vi "SubMenu.vi"(4 "ContextMenu":bool, 6 "SubMenu":bool, 7 "User Event":refnum<user-event>, 8 "error in (no error)":errorcluster, 9 "Tag":string, 10 "Selected Area":T2, 11 "Menu in":refnum<class "Menu.lvclass">) -> (0 "error out":errorcluster, 3 "Menu out":refnum<class "Menu.lvclass">)   [LabVIEW 2021, in "Menu.lvlib" / "Menu.lvclass"]
uses:
  Menu.lvclass
  <vilib>/Utility/miscctls.llb/LVPoint32TypeDef.ctl
  <vilib>/Utility/miscctls.llb/LVRectTypeDef.ctl
  <vilib>/event_ctls.llb/usereventprio.ctl
  UIShadow/src/Shadow.lvclass
  <vilib>/Utility/miscctls.llb/LVPositionTypeDef.ctl
  MenuSelection.ctl
  dc479f3e-3cf5-4ae2-bb41-5e206b11c71e.vi
  GetBackgroundColor.vi
  GetDVR.vi
  Picture2D/src/Color/Color.lvclass
  Menu.lvclass/Menu.ctl
  FrontPanel/src/FrontPanel.lvlib
panel:
  in  "Coords":T1
  in  "CtrlRef":refnum<vi>
  in  "notifier":refnum<notifier>
  out "Selected Area":T2
  out "Selected Tag":string
  out "Picture":picture
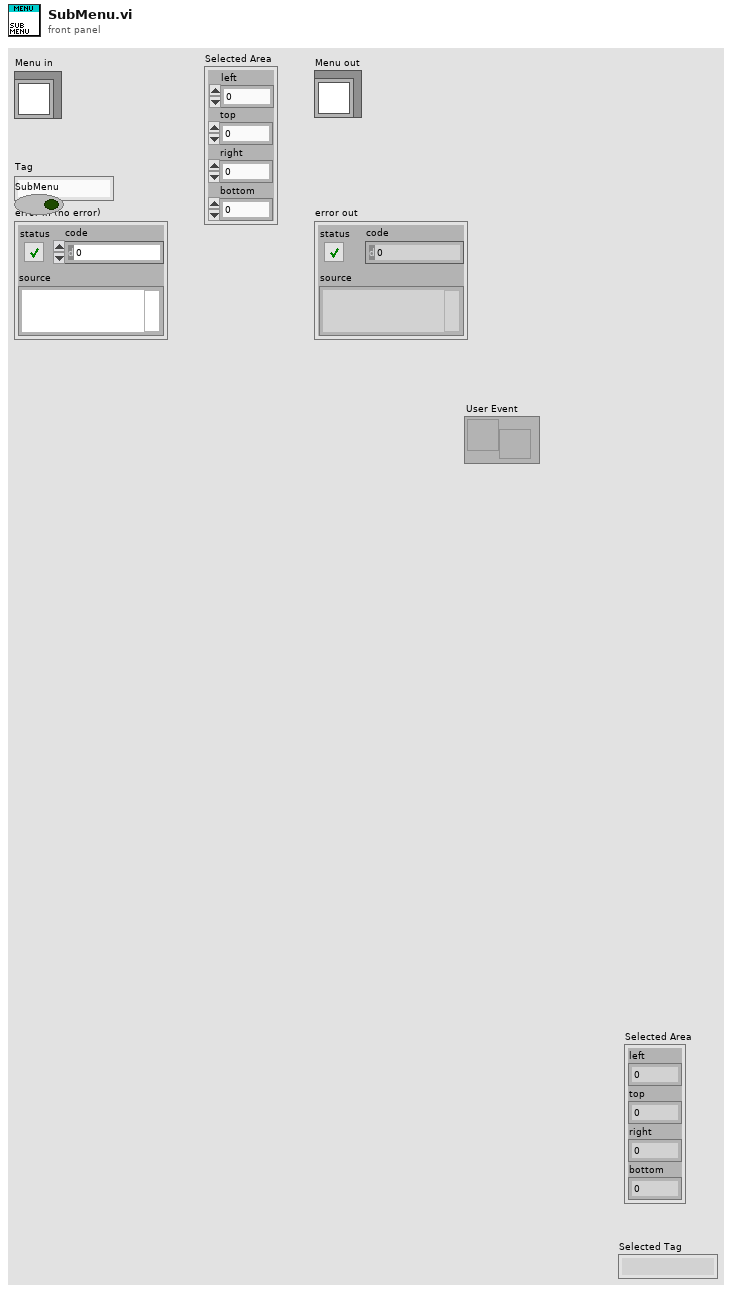
[diagram p1: front panel]
types:
  T1 = typedef "LVPoint32TypeDef.ctl" = cluster{"Horizontal":i32, "Vertical":i32}
  T2 = cluster{"left":i16, "top":i16, "right":i16, "bottom":i16}
  T3 = typedef "LVRectTypeDef.ctl" = cluster{"Left":i16, "Top":i16, "Right":i16, "Bottom":i16}
  T4 = typedef "usereventprio.ctl" = enum32{"high priority", "normal priority"}
  T5 = typedef "LVPositionTypeDef.ctl" = cluster{"Left":i32, "Top":i32}
  T6 = typedef "Menu.lvlib/Menu.lvclass/MenuSelection.ctl" = cluster{"ItemTag":string, "ItemPath":string}
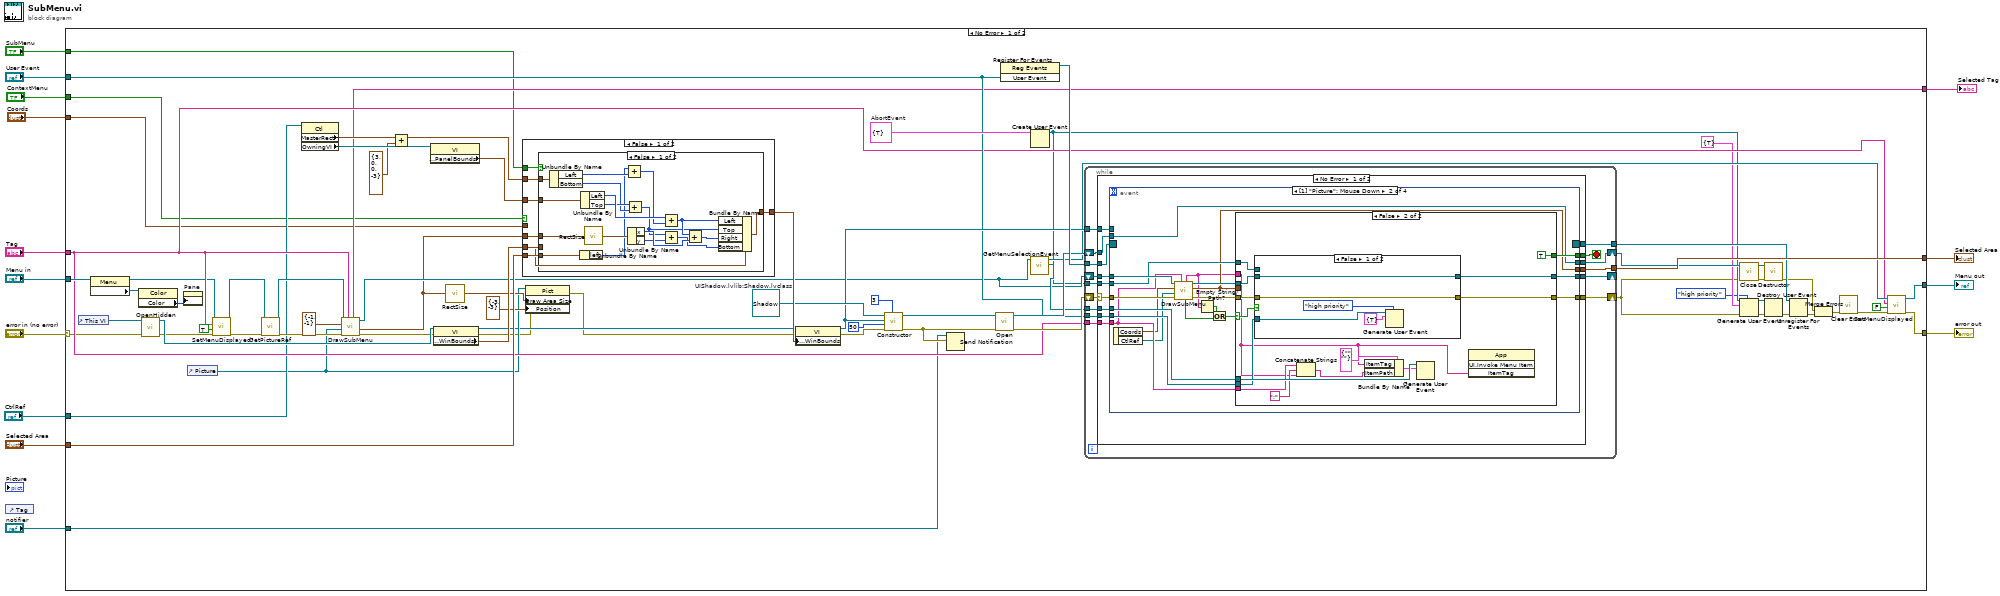
[diagram p0: block diagram]
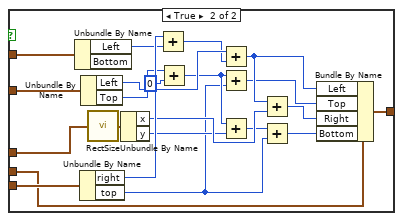
[diagram p2: hidden frame]
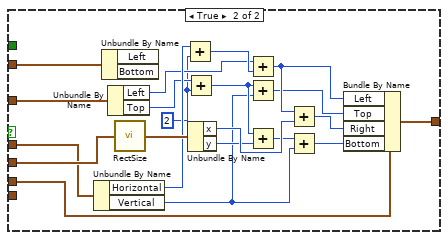
[diagram p3: hidden frame]
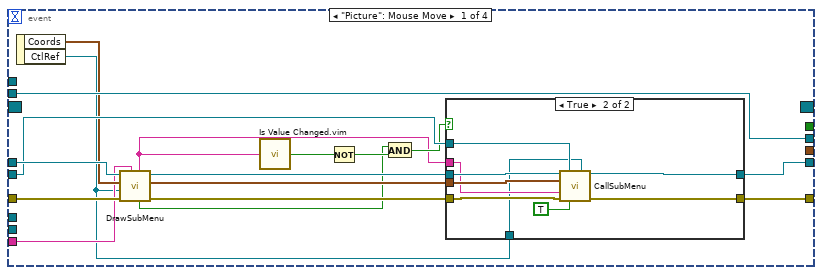
[diagram p4: hidden frame]
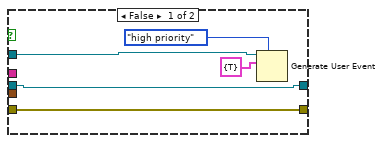
[diagram p5: hidden frame]
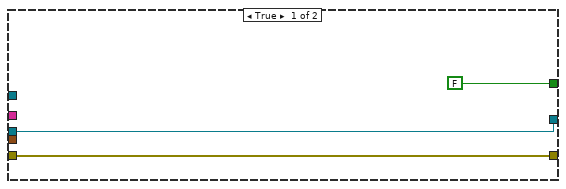
[diagram p6: hidden frame]
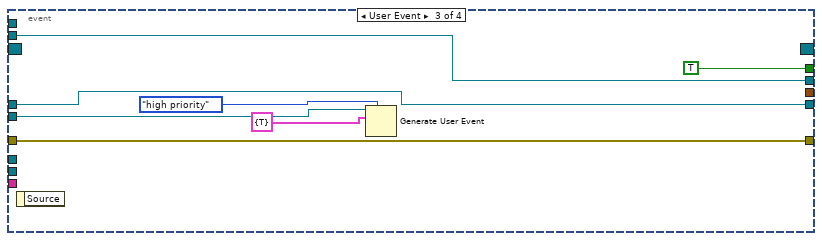
[diagram p8: hidden frame]
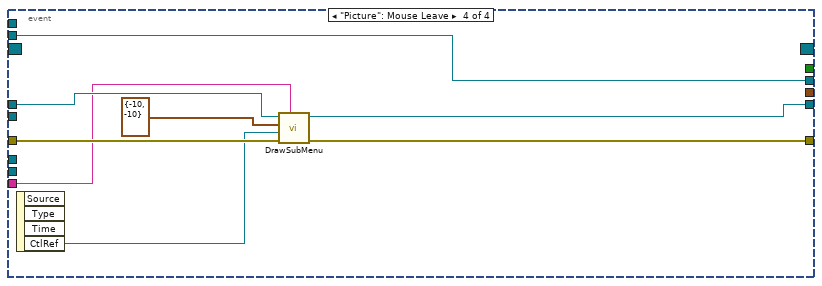
[diagram p9: hidden frame]
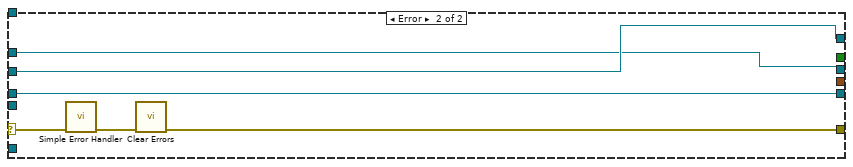
[diagram p10: hidden frame]
diagram:
  n1 = control-ref of="Tag"() -> ()  [unwired: 1 out]
  n2 = case shown="No Error" "error in (no error)" {
    selector: "error in (no error)" -> [w42 w281]
    tunnel: "Selected Area" -> [w84 _]
    tunnel: [w77 _] -> w13
    tunnel: "SubMenu" -> [w28 _]
    tunnel: "User Event" -> [w58 _]
    tunnel: "Menu in" -> [w55 w282]
    tunnel: [w51 w282] -> w9
    tunnel: "Tag" -> [w50 _]
    tunnel: [w48 w281] -> w7
    tunnel: "notifier" -> [w30 _]
    tunnel: [w29 _] -> w4
    tunnel: "CtrlRef" -> [w23 _]
    tunnel: "ContextMenu" -> [w21 _]
    tunnel: "Coords" -> [w20 _]
    frame No Error {
      w70 = refnum<class "Shadow.lvclass"> refnum  # UIShadow.lvlib:Shadow.lvclass
      w74 = cluster{"Abort":bool} {"Abort"=TRUE}  # AbortEvent
      n3 = control-ref of="This VI"() -> (w68:refnum<vi>)
      n4 = property class="Menu"(reference=w55) -> (reference out=w26:refnum<class "Menu.lvclass">, "Public:Background Color"=w25:refnum<class "Color.lvclass">)  [unwired: 1 in, 1 out]
      n5 = property class="Color"(reference=w25) -> ("Color"=w24:u32)  [unwired: 1 in, 2 out]
      n6 = call "OpenHidden.vi"("error in (no error)"=w42, "VI in"=w68) -> ("error out"=w41:errorcluster, "VI out"=w85:refnum<vi>)  [unwired: 8 in]
      n7 = property on="Pane" class="Pane"("PaneColor"=w24) -> ()  [unwired: 2 in, 2 out]
      n8 = control-ref of="Picture"() -> (w22:refnum<vi>)
      n9 = call "SetMenuDisplayed.vi"("error in (no error)"=w41, "Displayed"=TRUE, "Tag"=w50, "Menu in"=w26) -> ("error out"=w47:errorcluster, "Menu out"=w46:refnum<class "Menu.lvclass">)  [unwired: 6 in]
      n10 = call "GetPictureRef.vi"("error in (no error)"=w47, "Menu in"=w46) -> ("error out"=w44:errorcluster, "Menu out"=w45:refnum<class "Menu.lvclass">)  [unwired: 7 in, 1 out]
      n11 = property class="Ctl"(reference=w23) -> ("MasterRect"=w83:T3, "OwningVI"=w82:refnum<vi>)  [unwired: 1 in, 2 out]
      n12 = call "DrawSubMenu.vi"("Tag"=w50, "error in (no error)"=w44, "Pict Refnum"=w22, "Coords"=T1 {"Horizontal"=-1, "Vertical"=-1}, "Menu in"=w45) -> ("error out"=w43:errorcluster, "Global Area"=w27:T2, "Menu out"=w56:refnum<class "Menu.lvclass">, "Selected Tag"=w29:string)  [unwired: 1 in, 2 out]
      n13 = Add(x=w83, y=T3 {"Left"=3, "Top"=0, "Right"=0, "Bottom"=-3}) -> (x+y=w19:T3)
      n14 = property class="VI"(reference=w82) -> ("Front Panel.PanelBounds"=w81:T3)  [unwired: 1 in, 2 out]
      n15 = property class="VI"(reference=w85, error in=w43) -> (reference out=w17:refnum<vi>, error out=w16:errorcluster, "Front Panel.WinBounds"=w78:T3)
      n16 = call <vilib>:"RectSize.vi"("rect"=w27) -> ("point"=w76:cluster{"x":i16, "y":i16})
      n17 = case shown="False" w21 {
        tunnel: w84 -> [w92 _]
        tunnel: w19 -> [w91 w154]
        tunnel: w81 -> [w90 w153]
        tunnel: [w89 w152] -> w79
        tunnel: w78 -> [w88 w151]
        tunnel: w28 -> [w87 _]
        tunnel: w27 -> [w86 w150]
        tunnel: w20 -> [_ w136]
        frame False {
          n18 = case shown="False" w87 {
            tunnel: w92 -> [w110 w132]
            tunnel: w91 -> [w99 w120]
            tunnel: w90 -> [w98 w119]
            tunnel: [w96 w118] -> w89
            tunnel: w88 -> [w95 w117]
            tunnel: w86 -> [w94 w116]
            frame False {
              n19 = Unbundle By Name(w99) -> ("Left"=w100:i16, "Bottom"=w97:i16)
              n20 = Unbundle By Name(w110) -> ("left"=w93:i16)
              n21 = Unbundle By Name(w98) -> ("Left"=w109:i16, "Top"=w108:i16)
              n22 = call <vilib>:"RectSize.vi"("rect"=w94) -> ("point"=w111:cluster{"x":i16, "y":i16})
              n23 = Add(x=w93, y=w100) -> (x+y=w101:i16)
              n24 = Add(x=w108, y=w97) -> (x+y=w102:i16)
              n25 = Unbundle By Name(w111) -> ("x"=w106:i16, "y"=w103:i16)
              n26 = Add(x=w109, y=w101) -> (x+y=w107:i16)
              n27 = Add(x=w102, y=w103) -> (x+y=w104:i16)
              n28 = Add(x=w107, y=w106) -> (x+y=w105:i16)
              n29 = Bundle By Name(cluster=w95, "Left"=w107, "Top"=w102, "Right"=w105, "Bottom"=w104) -> (w96:T3)
            }
            frame True {
              n30 = Unbundle By Name(w120) -> ("Left"=w121:i16)  [unwired: 1 out]
              n31 = Unbundle By Name(w132) -> ("right"=w130:i16, "top"=w113:i16)
              n32 = Unbundle By Name(w119) -> ("Left"=w131:i16, "Top"=w129:i16)
              n33 = call <vilib>:"RectSize.vi"("rect"=w116) -> ("point"=w133:cluster{"x":i16, "y":i16})
              n34 = Unbundle By Name(w133) -> ("x"=w127:i16, "y"=w124:i16)
              n35 = Add(x=w130, y=w121) -> (x+y=w122:i16)
              n36 = Add(x=w129, y=i16 0) -> (x+y=w123:i16)
              n37 = Add(x=w131, y=w122) -> (x+y=w128:i16)
              n38 = Add(x=w123, y=w113) -> (x+y=w115:i16)
              n39 = Add(x=w123, y=w124) -> (x+y=w125:i16)
              n40 = Add(x=w128, y=w127) -> (x+y=w126:i16)
              n41 = Add(x=w125, y=w113) -> (x+y=w114:i16)
              n42 = Bundle By Name(cluster=w117, "Left"=w128, "Top"=w115, "Right"=w126, "Bottom"=w114) -> (w118:T3)
            }
          }
        }
        frame True {
          w134 = i16 2 ("y")
          n43 = Unbundle By Name(w136) -> ("Horizontal"=w148:i32, "Vertical"=w137:i32)
          n44 = Unbundle By Name(w154) -> ()  [unwired: 2 out]
          n45 = Unbundle By Name(w153) -> ("Left"=w135:i16, "Top"=w147:i16)
          n46 = call <vilib>:"RectSize.vi"("rect"=w150) -> ("point"=w149:cluster{"x":i16, "y":i16})
          n47 = Add(x=w148, y=w134) -> (x+y=w140:i32)
          n48 = Add(x=w147, y=w134) -> (x+y=w141:i16)
          n49 = Unbundle By Name(w149) -> ("x"=w145:i16, "y"=w142:i16)
          n50 = Add(x=w135, y=w140) -> (x+y=w146:i32)
          n51 = Add(x=w141, y=w137) -> (x+y=w139:i32)
          n52 = Add(x=w141, y=w142) -> (x+y=w143:i16)
          n53 = Add(x=w146, y=w145) -> (x+y=w144:i32)
          n54 = Add(x=w143, y=w137) -> (x+y=w138:i32)
          n55 = Bundle By Name(cluster=w151, "Left"=w146, "Top"=w139, "Right"=w144, "Bottom"=w138) -> (w152:T3)
        }
      }
      n56 = property class="Pict"(reference=w22, error in=w16, "Draw Area Size"=w76, "Position"=T5 {"Left"=-3, "Top"=-3}) -> (error out=w15:errorcluster)  [unwired: 1 out]
      n57 = property class="VI"(reference=w17, error in=w15, "Front Panel.WinBounds"=w79) -> (reference out=w62:refnum<vi>, error out=w65:errorcluster)
      n58 = call "Constructor.vi"("Offset"=i16 3, "error in (no error)"=w65, "Transparancy"=50, "VI Refnum"=w62, "Shadow in"=w70) -> ("error out"=w31:errorcluster, "Shadow out"=w64:refnum<class "Shadow.lvclass">)  [unwired: 5 in]
      n59 = Send Notification(notification=w31, notifier=w30) -> ()  [unwired: 1 in, 2 out]
      n60 = call "Open.vi"("error in (no error)"=w31, "Shadow in"=w64) -> ("error out"=w66:errorcluster, "Shadow out"=w63:refnum<class "Shadow.lvclass">)  [unwired: 8 in]
      n61 = register-events(w58) -> (reference out=w73:refnum<event-registration>)  [unwired: 2 in, 1 out]
      n62 = call "GetMenuSelectionEvent.vi"("Menu in"=w56) -> ("MenuSelectionEvent"=w57:refnum<user-event>, "Menu out"=w52:refnum<class "Menu.lvclass">)  [unwired: 8 in, 1 out]
      n63 = Create User Event(user event datatype=w74) -> (user event=w36:refnum<user-event>)  [unwired: 1 in, 1 out]
      n64 = while {
        shift-right: [w168] -> w60
        shift-left: w63 -> [w169]
        shift-right: [w166] -> w34
        shift-left: w66 -> [w167]
        shift-right: [w164] -> _
        shift-left: w56 -> [w165]
        tunnel: w50 -> [w163]
        tunnel: w57 -> [w162]
        tunnel: [w160] -> w77
        tunnel: w73 -> [w159]
        tunnel: [w158] -> w71
        tunnel: w36 -> [w157]
        tunnel: w62 -> [w156]
        tunnel: w58 -> [w155]
        stop <- w161 stop-if-true
        n65 = case shown="No Error" w167 {
          selector: w167 -> [w182 w280]
          tunnel: w169 -> [w184 w276]
          tunnel: [w183 w276] -> w168
          tunnel: [w181 w278] -> w166
          tunnel: w165 -> [w180 w275]
          tunnel: [w179 w275] -> w164
          tunnel: w163 -> [w178 _]
          tunnel: w162 -> [w177 _]
          tunnel: [w176 _] -> w161
          tunnel: [w175 _] -> w160
          tunnel: w159 -> [w174 w277]
          tunnel: [w173 w277] -> w158
          tunnel: w157 -> [w172 _]
          tunnel: w156 -> [w171 _]
          tunnel: w155 -> [w170 _]
          frame No Error {
            n66 = event shown="[1] \"Picture\": Mouse Down" {
              selector: w174 -> [_ _ _ _]
              dyn-events: [_ _ _ _] -> w173
              timeout: _ -> [_ _ _ _]
              tunnel: w184 -> [w200 w221 w266 w271]
              tunnel: [w200 w221 w266 w271] -> w183
              tunnel: [w197 w227 w263 w269] -> w181
              tunnel: w182 -> [w199 w231 w263 w270]
              tunnel: w180 -> [w201 w234 w264 w274]
              tunnel: [w195 w229 w264 w273] -> w179
              tunnel: w178 -> [w189 w224 _ w267]
              tunnel: w177 -> [_ w233 _ _]
              tunnel: [_ w232 TRUE _] -> w176
              tunnel: [_ w220 _ _] -> w175
              tunnel: w172 -> [w194 w226 w262 _]
              tunnel: w171 -> [_ _ _ _]
              tunnel: w170 -> [_ w225 _ _]
              event "Picture": Mouse Move {
                n67 = event-data() -> ("Coords"=w190:T1, "CtlRef"=w185:refnum<vi>)  [unwired: 1 in]
                n68 = call "DrawSubMenu.vi"("Tag"=w189, "error in (no error)"=w199, "Pict Refnum"=w185, "Coords"=w190, "Menu in"=w201) -> ("error out"=w198:errorcluster, "Selected Area"=w187:T2, "Menu out"=w196:refnum<class "Menu.lvclass">, "SubMenu"=w186:bool, "Selected Tag"=w188:string)  [unwired: 1 in, 1 out]
                n69 = call "Is Value Changed.vim"("value"=w188) -> ("changed or first call?"=w191:bool)
                n70 = Not(x=w191) -> (.not. x?=w192:bool)
                n71 = And(x=w186, y=w192) -> (x .and. y?=w193:bool)
                n72 = case shown="True" w193 {
                  tunnel: w187 -> [_ w210]
                  tunnel: w196 -> [w206 w214]
                  tunnel: [w206 w213] -> w195
                  tunnel: w188 -> [_ w209]
                  tunnel: w198 -> [w202 w211]
                  tunnel: [w202 w212] -> w197
                  tunnel: w194 -> [w203 w215]
                  tunnel: w185 -> [_ w207]
                  frame False {
                    n73 = Generate User Event(priority (normal)=usereventprio."high priority", user event=w203, event data cluster=cluster{"Abort":bool} {"Abort"=TRUE} ("event data")) -> ()  [unwired: 1 in, 2 out]
                  }
                  frame True {
                    n74 = call "CallSubMenu.vi"("Menu in"=w214, "User Event"=w215, "CtrlRef"=w207, "Selected Area"=w210, "Selected Tag"=w209, "error in (no error)"=w211, "SubMenu"=TRUE) -> ("Menu out"=w213:refnum<class "Menu.lvclass">, "error out"=w212:errorcluster)  [unwired: 7 in]
                  }
                }
              }
              event "Picture": Mouse Down {
                n75 = event-data() -> ("Coords"=w223:T1, "CtlRef"=w222:refnum<vi>)  [unwired: 1 in]
                n76 = call "DrawSubMenu.vi"("Tag"=w224, "error in (no error)"=w231, "Pict Refnum"=w222, "Coords"=w223, "Menu in"=w234) -> ("error out"=w228:errorcluster, "Selected Area"=w220:T2, "Menu out"=w230:refnum<class "Menu.lvclass">, "SubMenu"=w218:bool, "Selected Tag"=w216:string)  [unwired: 1 in, 1 out]
                n77 = Empty String/Path?(string/path=w216) -> (empty?=w217:bool)
                n78 = Or(x=w217, y=w218) -> (x .or. y?=w219:bool)
                n79 = case shown="False" w219 {
                  selector: w219 -> [_ w240]
                  tunnel: w233 -> [_ w252]
                  tunnel: [FALSE TRUE] -> w232
                  tunnel: w230 -> [w236 w246]
                  tunnel: [w236 w245] -> w229
                  tunnel: w228 -> [w235 w244]
                  tunnel: [w235 w243] -> w227
                  tunnel: w226 -> [_ w242]
                  tunnel: w225 -> [_ w241]
                  tunnel: w224 -> [_ w239]
                  tunnel: w220 -> [_ _]
                  tunnel: w216 -> [_ w238]
                  frame True {
                  }
                  frame False {
                    n80 = case shown="False" w240 {
                      tunnel: w246 -> [w257 w259]
                      tunnel: [w257 w259] -> w245
                      tunnel: w244 -> [w256 w258]
                      tunnel: [w256 w258] -> w243
                      tunnel: w242 -> [_ _]
                      tunnel: w241 -> [w254 _]
                      frame False {
                        n81 = Generate User Event(priority (normal)=usereventprio."high priority", user event=w254, event data cluster=cluster{"Abort":bool} {"Abort"=TRUE} ("event data")) -> ()  [unwired: 1 in, 2 out]
                      }
                      frame True {
                      }
                    }
                    n82 = Concatenate Strings(w239, ":" ("string"), w238) -> (w249:string)
                    n83 = Bundle By Name(cluster=T6 {"ItemTag"="", "ItemPath"=""} ("event data"), "ItemTag"=w238, "ItemPath"=w249) -> (w250:T6)
                    n84 = Generate User Event(user event=w252, event data cluster=w250) -> ()  [unwired: 2 in, 2 out]
                    n85 = invoke class="App" method="UI.Invoke Menu Item"("ItemTag"=w238) -> ()  [unwired: 3 in, 4 out]
                  }
                }
              }
              event User Event {
                n86 = event-data() -> ()  [unwired: 1 in, 1 out]
                n87 = Generate User Event(priority (normal)=usereventprio."high priority", user event=w262, event data cluster=cluster{"Abort":bool} {"Abort"=TRUE}) -> ()  [unwired: 1 in, 2 out]
              }
              event "Picture": Mouse Leave {
                n88 = event-data() -> ("CtlRef"=w268:refnum<vi>)  [unwired: 1 in, 3 out]
                n89 = call "DrawSubMenu.vi"("Tag"=w267, "error in (no error)"=w270, "Pict Refnum"=w268, "Coords"=T1 {"Horizontal"=-10, "Vertical"=-10}, "Menu in"=w274) -> ("error out"=w269:errorcluster, "Menu out"=w273:refnum<class "Menu.lvclass">)  [unwired: 1 in, 4 out]
              }
            }
          }
          frame Error {
            n90 = call <vilib>:"Simple Error Handler.vi"("error in (no error)"=w280) -> ("error out"=w279:errorcluster)  [unwired: 4 in, 4 out]
            n91 = call <vilib>:"Clear Errors.vi"("error in (no error)"=w279) -> ("error out"=w278:errorcluster)  [unwired: 5 in, 1 out]
          }
        }
      }
      n92 = call "Close.vi"("error in (no error)"=w34, "Shadow in"=w60) -> ("error out"=w61:errorcluster, "Shadow out"=w59:refnum<class "Shadow.lvclass">)  [unwired: 8 in]
      n93 = Generate User Event(priority (normal)=usereventprio."high priority", user event=w36, event data cluster=cluster{"Abort":bool} {"Abort"=TRUE} ("event data"), error in=w34) -> (user event out=w35:refnum<user-event>, error out=w33:errorcluster)
      n94 = call "Destructor.vi"("error in (no error)"=w61, "Shadow in"=w59) -> ("error out"=w49:errorcluster)  [unwired: 9 in]
      n95 = Destroy User Event(user event=w35, error in=w33) -> (error out=w72:errorcluster)
      n96 = Unregister For Events(event registration refnum=w71, error in=w72) -> (error out=w39:errorcluster)
      n97 = Merge Errors(w49, w39) -> (w40:errorcluster)
      n98 = call <vilib>:"Clear Errors.vi"("error in (no error)"=w40) -> ("error out"=w38:errorcluster)  [unwired: 5 in, 1 out]
      n99 = call "SetMenuDisplayed.vi"("error in (no error)"=w38, "Displayed"=FALSE, "Tag"=w50, "Menu in"=w52) -> ("error out"=w48:errorcluster, "Menu out"=w51:refnum<class "Menu.lvclass">)  [unwired: 6 in]
    }
    frame Error {
    }
  }
  "Selected Tag" <- w4
  "Selected Area" <- w13
  "error out" <- w7
  "Menu out" <- w9
